vi "Monkey Died.vi"(8 "error in (no error)":errorcluster, 10 "Monkey ID":string, 11 "Tamer in":refnum<class "Tamer.lvclass">) -> (0 "error out":errorcluster, 3 "Tamer out":refnum<class "Tamer.lvclass">)   [LabVIEW 2020, in "CIRCUS_uServices.lvlib" / "Tamer.lvlib" / "Tamer.lvclass"]
uses:
  Tamer.lvclass
  Tamer.lvclass/Tamer.ctl
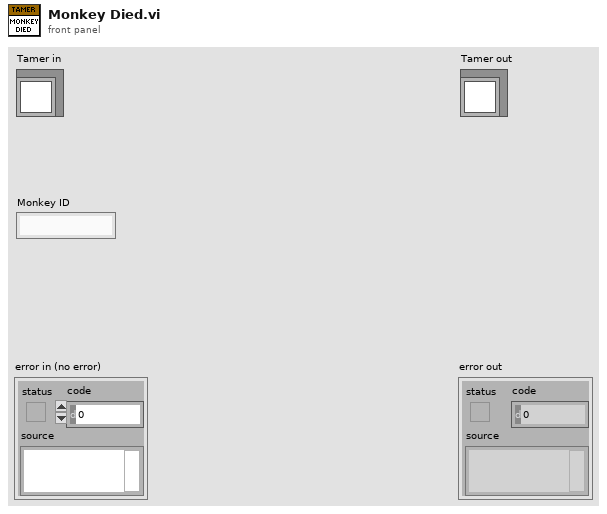
[diagram p1: front panel]
types:
  T1 = typedef "CIRCUS_uServices.lvlib/Run Utilities.lvlib/Synchronize FPGA Cluster.ctl" = cluster{"Status":bool, "FPGA Name":string}
  T2 = typedef "CIRCUS_uServices.lvlib/Run Utilities.lvlib/Monkey Status.ctl" = enum16{"Init", "Paused", "Ongoing", "Stopped", "Finished (no errors)", "Finished (with errors)"}
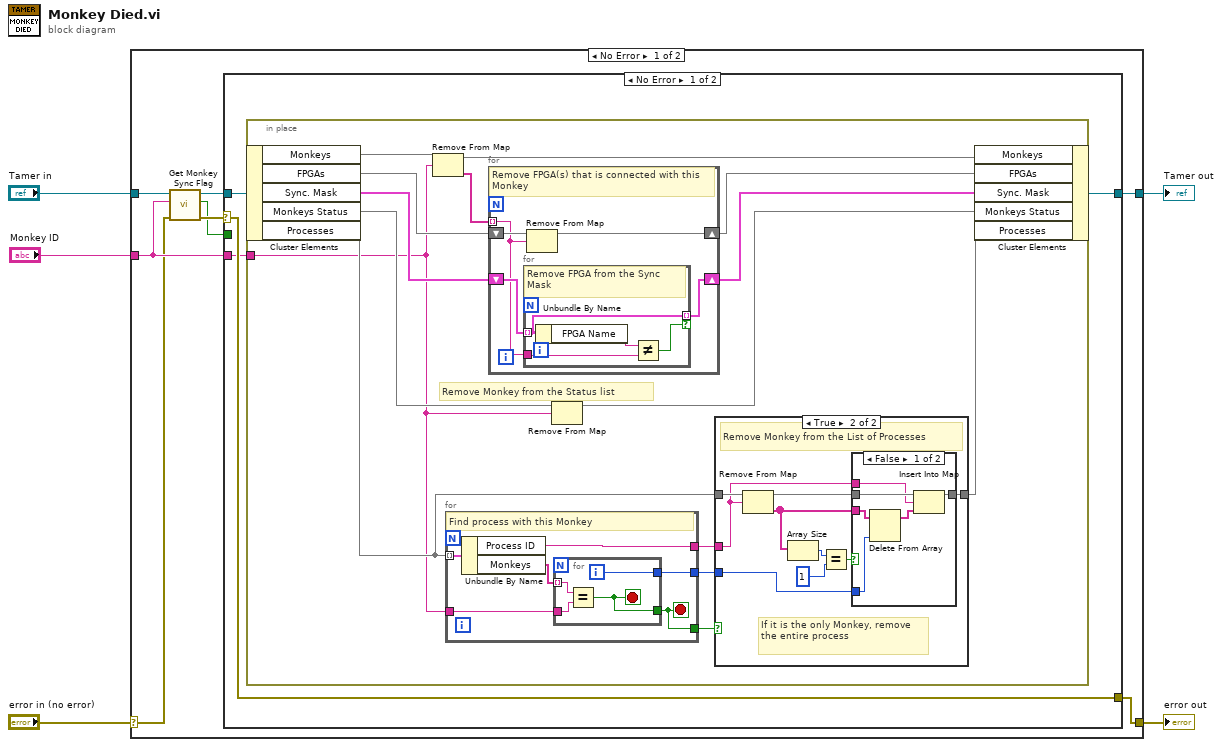
[diagram p0: block diagram]
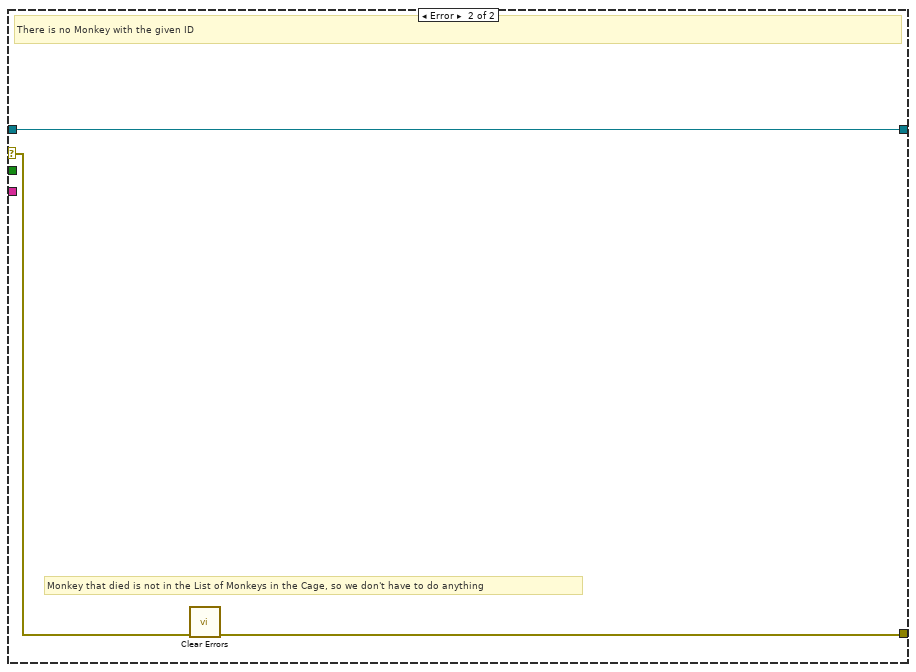
[diagram p4: hidden frame]
diagram:
  n1 = case shown="No Error" "error in (no error)" {
    selector: "error in (no error)" -> [w10 w73]
    tunnel: [w8 w73] -> w4
    tunnel: [w7 w72] -> w2
    tunnel: "Tamer in" -> [w13 w72]
    tunnel: "Monkey ID" -> [w11 _]
    frame No Error {
      n2 = call-dynamic "Get Monkey Sync Flag.vi"("error in (no error)"=w10, "Monkey ID"=w11, "Tamer in"=w13) -> ("error out"=w9:errorcluster, "Monkey Sync Flag"=w6:bool, "Tamer out"=w12:refnum<class "Tamer.lvclass">)  [unwired: 6 in]
      n3 = case shown="No Error" w9 {
        selector: w9 -> [w17 w70]
        tunnel: w12 -> [w16 w71]
        tunnel: w11 -> [w15 _]
        tunnel: [w17 w69] -> w8
        tunnel: [w14 w71] -> w7
        tunnel: w6 -> [_ _]
        frame No Error {
          n4 = in-place {
            in-place-border: w15 -> [w18]
            # "Remove Monkey from the Status list"
            n5 = in-place-cluster #1(w16) -> ("Monkeys"=w28:map{string, string[]}, "FPGAs"=w27:map{string, string}, "Sync. Mask"=w26:T1[], "Monkeys Status"=w25:map{string, T2}, "Processes"=w24:map{string, string[]})
            n6 = Remove From Map(10:w18, 11:w28) -> (1:w30:string[], 3:w19:map{string, string[]})  [unwired: 1 out]
            n7 = for {
              tunnel: w24 -> [w64] mode=indexing
              tunnel: w18 -> [w62]
              tunnel: [w61] -> w31
              tunnel: [w60] -> w32
              tunnel: [w59] -> w29
              stop <- w59 stop-if-true
              # "Find process with this Monkey"
              n8 = Unbundle By Name(w64) -> ("Process ID"=w61:string, "Monkeys"=w63:string[])
              n9 = for {
                tunnel: w63 -> [w68] mode=indexing
                tunnel: w62 -> [w67]
                tunnel: [w66] -> w59
                tunnel: [w65] -> w60
                i -> [w65]
                stop <- w66 stop-if-true
                n10 = Equal?(x=w68, y=w67) -> (x = y?=w66:bool)
              }
            }
            n11 = for {
              tunnel: w30 -> [w51] mode=indexing
              shift-right: [w53] -> w20
              shift-left: w27 -> [w54]
              shift-right: [w50] -> w21
              shift-left: w26 -> [w52]
              # "Remove FPGA(s) that is connected with this Monkey"
              n12 = for {
                tunnel: w52 -> [w56] mode=indexing
                tunnel: w51 -> [w57]
                tunnel: [w56] -> w50 mode=indexing if=w55
                # "Remove FPGA from the Sync Mask"
                n13 = Unbundle By Name(w56) -> ("FPGA Name"=w58:string)
                n14 = Not Equal?(x=w58, y=w57) -> (x != y?=w55:bool)
              }
              n15 = Remove From Map(10:w51, 11:w54) -> (3:w53:map{string, string})  [unwired: 2 out]
            }
            n16 = Remove From Map(10:w18, 11:w25) -> (3:w22:map{string, T2})  [unwired: 2 out]
            n17 = case shown="True" w29 {
              tunnel: w24 -> [w33 w42]
              tunnel: w32 -> [_ w36]
              tunnel: w31 -> [_ w35]
              tunnel: [w33 w34] -> w23
              frame False {
                # "This Monkey is not present in the List of Processes"
              }
              frame True {
                # "If it is the only Monkey, remove the entire process"
                # "Remove Monkey from the List of Processes"
                n18 = Remove From Map(10:w35, 11:w42) -> (1:w37:string[], 3:w38:map{string, string[]})  [unwired: 1 out]
                n19 = Array Size(array=w37) -> (size(s)=w41:i32)
                n20 = Equal?(x=w41, y=1) -> (x = y?=w39:bool)
                n21 = case shown="False" w39 {
                  tunnel: w38 -> [w46 w49]
                  tunnel: [w43 w49] -> w34
                  tunnel: w37 -> [w48 _]
                  tunnel: w36 -> [w47 _]
                  tunnel: w35 -> [w45 _]
                  frame False {
                    n22 = Delete From Array(array=w48, index=w47) -> (array with subset deleted=w44:string[])  [unwired: 1 in, 1 out]
                    n23 = Insert Into Map(map in=w46, key=w45, value=w44) -> (map out=w43:map{string, string[]})  [unwired: 2 out]
                  }
                  frame True {
                  }
                }
              }
            }
            n24 = in-place-cluster #1("Monkeys"=w19, "FPGAs"=w20, "Sync. Mask"=w21, "Monkeys Status"=w22, "Processes"=w23) -> (w14:refnum<class "Tamer.lvclass">)
          }
        }
        frame Error {
          # "Monkey that died is not in the List of Monkeys in the Cage, so we don't have to do anything"
          # "There is no Monkey with the given ID"
          n25 = call <vilib>:"Clear Errors.vi"("error in (no error)"=w70) -> ("error out"=w69:errorcluster)  [unwired: 5 in, 1 out]
        }
      }
    }
    frame Error {
    }
  }
  "error out" <- w4
  "Tamer out" <- w2
